vi "Pin Map Client FGV.vi"(8 "error in":errorcluster, 11 "action":T2) -> (0 "error out":errorcluster, 3 "grpc client id":T1)   [LabVIEW 2020, in "MeasurementLink Pin Map Client Wrapper.lvlib"]
uses:
  MeasurementLink Pin Map Client Wrapper.lvlib
  Action.ctl
  <vilib>/gRPC/LabVIEW gRPC Library/Shared/grpcId.ctl
  MeasurementLink Discovery Client/RPC Messages/ni_measurementlink_discovery_v1_ResolveServiceRequest.ctl
  <vilib>/gRPC/LabVIEW gRPC Library/grpc-lvsupport-release.lvlib
  MeasurementLink Discovery Client Wrapper/MeasurementLink Discovery Client Wrapper.lvlib
  MeasurementLink Discovery Client/MeasurementLink Discovery Client.lvlib
  MeasurementLink Pin Map Client/MeasurementLink Pin Map Client.lvlib
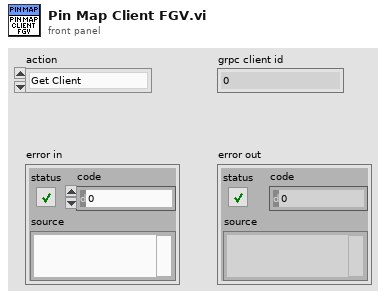
[diagram p1: front panel]
types:
  T1 = typedef "grpc-lvsupport-release.lvlib/grpcId.ctl" = u64
  T2 = typedef "MeasurementLink Pin Map Client Wrapper.lvlib/Action.ctl" = enum16{"Get Client", "Destroy Client"}
  T3 = typedef "MeasurementLink Discovery Client.lvlib/ni_measurementlink_discovery_v1_ResolveServiceRequest.ctl" = cluster{"provided_interface":string, "service_class":string}
  T4 = typedef "MeasurementLink Discovery Client.lvlib/ni_measurementlink_discovery_v1_ServiceLocation.ctl" = cluster{"location":string, "insecure_port":string, "ssl_authenticated_port":string}
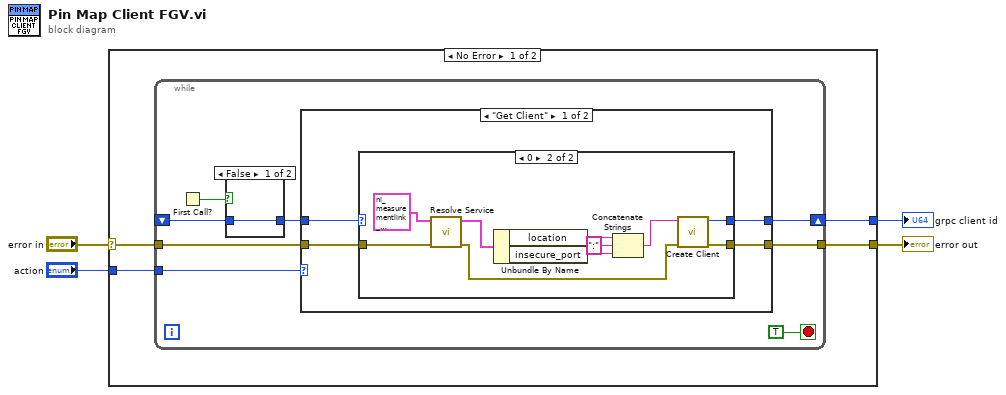
[diagram p0: block diagram]
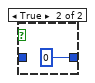
[diagram p2: hidden frame]
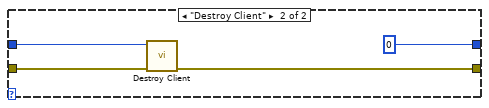
[diagram p4: hidden frame]
diagram:
  n1 = case shown="No Error" "error in" {
    selector: "error in" -> [w7 w39]
    tunnel: [w6 w39] -> w3
    tunnel: "action" -> [w8 _]
    tunnel: [w5 _] -> w1
    frame No Error {
      n2 = while {
        tunnel: w8 -> [w15]
        tunnel: w7 -> [w14]
        tunnel: [w13] -> w6
        shift-right: [w12] -> w5
        shift-left: _ -> [w10]
        stop <- TRUE stop-if-true
        n3 = First Call?() -> (First Call?: T/F=w11:bool)
        n4 = case shown="False" w11 {
          tunnel: w10 -> [w17 _]
          tunnel: [w17 T1 0 ("gRPC ID out")] -> w9
          frame False {
          }
          frame True {
          }
        }
        n5 = case shown="\"Get Client\"" w15 {
          tunnel: w14 -> [w19 w35]
          tunnel: [w22 w37] -> w13
          tunnel: [w21 T1 0 ("gRPC ID out")] -> w12
          tunnel: w9 -> [w20 w38]
          frame "Get Client" {
            n6 = case shown="0" w20 {
              selector: w20 -> [w24 _]
              tunnel: w19 -> [w23 w28]
              tunnel: [w23 w30] -> w22
              tunnel: [w24 w29] -> w21
              frame Default {
              }
              frame 0 {
                n7 = call "Resolve Service.vi"("error in"=w28, "request data"=T3 {"provided_interface"="ni.measurementlink.sessionmanagement.v1.SessionManagementService", "service_class"="ni.measurementlink.sessionmanagement.v1.SessionManagementService"}) -> ("error out"=w27:errorcluster, "response data"=w26:T4)  [unwired: 8 in]
                n8 = Unbundle By Name(w26) -> ("location"=w34:string, "insecure_port"=w33:string)
                n9 = Concatenate Strings(w34, ":" ("string"), w33) -> (w31:string)
                n10 = call "Create Client.vi"("error in"=w27, "address"=w31) -> ("error out"=w30:errorcluster, "gRPC ID Out"=w29:T1)  [unwired: 8 in]
              }
            }
          }
          frame "Destroy Client" {
            n11 = call "Destroy Client.vi"("error in"=w35, "gRPC ID"=w38) -> ("error out"=w37:errorcluster)  [unwired: 9 in]
          }
        }
      }
    }
    frame Error {
    }
  }
  "error out" <- w3
  "grpc client id" <- w1
